vi "Do.vi"(8 "error in (no error)":errorcluster, 10 "Actor in":refnum<class "Actor.lvclass">, 11 "Go Idle Msg":refnum<class "Go to Idle Msg.lvclass">) -> (0 "error out":errorcluster, 2 "Actor out":refnum<class "Actor.lvclass">)   [LabVIEW 2014, in "States.lvlib" / "Go to Idle Msg.lvclass"]
doc: "This VI delivers the message to the actor by calling the appropriate method(s) on the actor."
uses:
  Go to Idle Msg.lvclass
  <vilib>/ActorFramework/Actor/Actor.lvclass
  Process State/Process State.lvclass
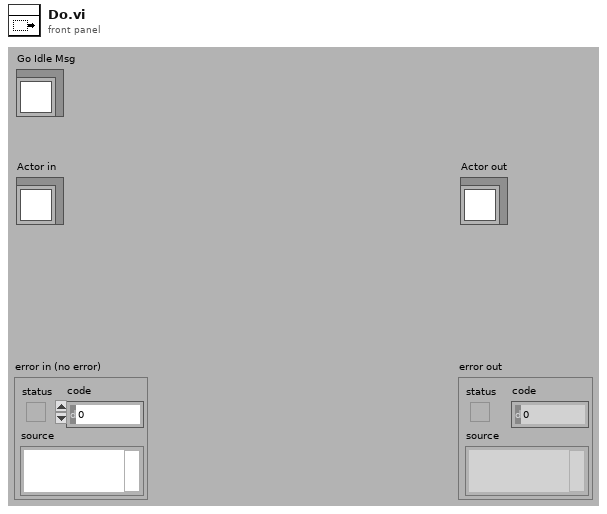
[diagram p1: front panel]
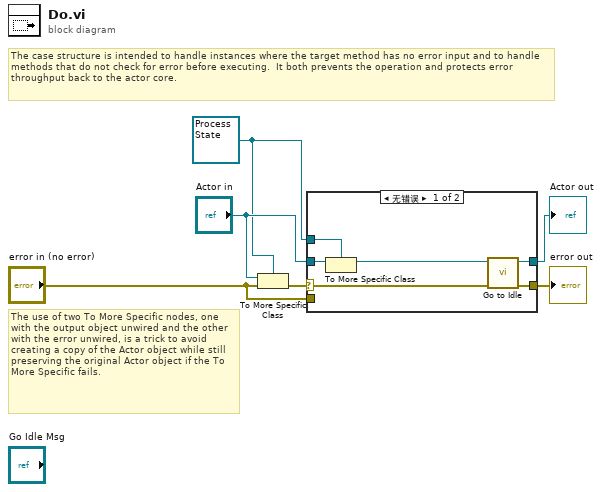
[diagram p0: block diagram]
diagram:
  w2 = refnum<class "Process State.lvclass"> refnum ("Actor in")
  # "The use of two To More Specific nodes, one with the output object unwired and the other with the error unwired, is a trick to avoid creating a copy of the Actor object while still preserving the original Actor object if the To More Specific fails."
  # "The case structure is intended to handle instances where the target method has no error input and to handle methods that do not check for error before executing.  It both prevents the operation and protects error throughput back to the actor core."
  n1 = To More Specific Class(target class=w2, reference="Actor in", error in="error in (no error)") -> (error out=w6:errorcluster)  [unwired: 1 out]
  n2 = case shown="无错误" w6 {
    selector: w6 -> [w10 _]
    tunnel: [w12 w13] -> w5
    tunnel: [w11 w14] -> w4
    tunnel: "Actor in" -> [w9 w14]
    tunnel: w2 -> [w8 _]
    tunnel: "error in (no error)" -> [_ w13]
    frame No Error {
      n3 = To More Specific Class(target class=w8, reference=w9) -> (specific class reference=w7:refnum<class "Process State.lvclass">)  [unwired: 1 in, 1 out]
      n4 = call-dynamic "Go to Idle.vi"("error in (no error)"=w10, "Process State in"=w7) -> ("error out"=w12:errorcluster, "Process State out"=w11:refnum<class "State Actor.lvclass">)  [unwired: 8 in]
    }
    frame Error {
      # "If type check fails, pass the original object out again."
    }
  }
  "error out" <- w5
  "Actor out" <- w4
